vi "Init.vi"(4 "Interlock message (\" -> Interlock!\")":string=" -> Interlock!", 6 "Name (SHV Name if empty)":string, 7 "Sample Containers SHV (Array!)":variant, 8 "error in (no error)":errorcluster, 9 "Stop Self on IL? (T)":bool=TRUE, 11 "Interlock Sample in":refnum<class "Interlock Sample.lvclass">) -> (0 "error out":errorcluster, 3 "Interlock Sample out":refnum<class "Interlock Sample.lvclass">)   [LabVIEW 2015, in "Interlocks.lvlib" / "Interlock Sample.lvclass"]
uses:
  Interlock Sample.lvclass
  Controls/Sample Container.ctl
  subs/Sample/Sample.lvclass
  Interlock Sample.lvclass/Interlock Sample.ctl
  Interlock/Interlock.lvclass/Interlock.ctl
  Interlock/Interlock.lvclass
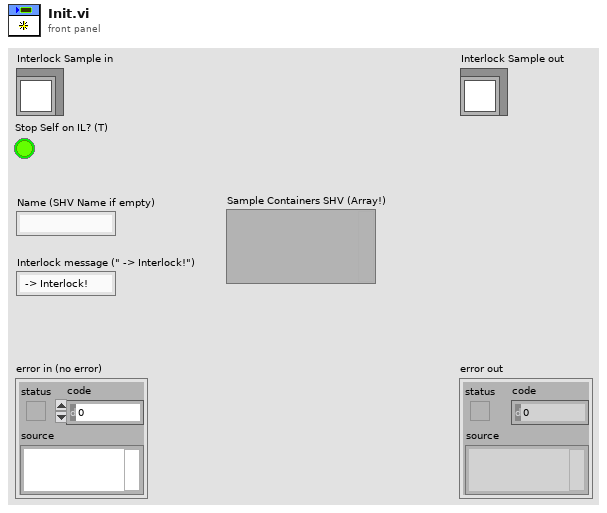
[diagram p1: front panel]
types:
  T1 = typedef "Sample Container.ctl" = cluster{"Sample In":refnum<k21>, "Sample Name":refnum<k21>, "Ti Cathode":refnum<k21>, "SampleQ":refnum<queue>}
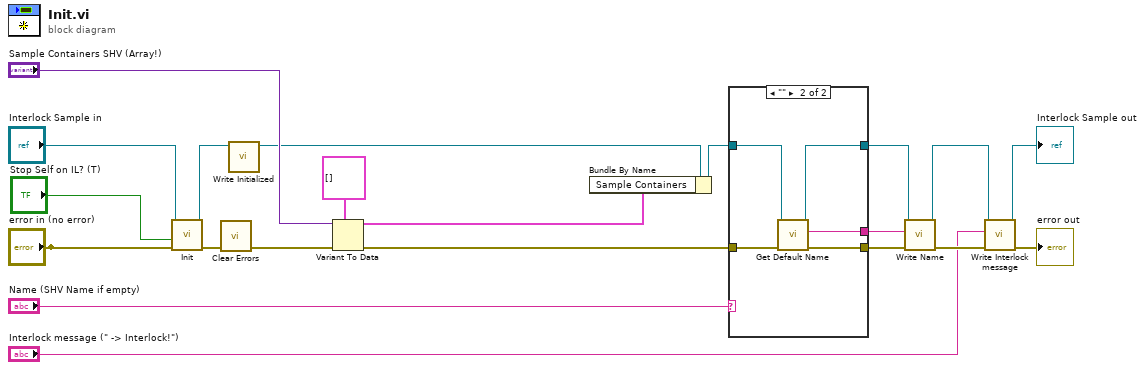
[diagram p0: block diagram]
diagram:
  n1 = call-parent "Init.vi"("error in (no error)"="error in (no error)", "Stop Self on IL? (T)"="Stop Self on IL? (T)", "Interlock in"="Interlock Sample in") -> ("error out"=w7:errorcluster, "Interlock out"=w4:refnum<class "Interlock Sample.lvclass">)  [unwired: 7 in]
  n2 = call <vilib>:"Clear Errors.vi"("error in (no error)"=w7) -> ()  [unwired: 5 in, 2 out]
  n3 = call-dynamic "Write Initialized.vi"("Interlock in"=w4) -> ("Interlock out"=w8:refnum<class "Interlock Sample.lvclass">)  [unwired: 10 in]
  n4 = Variant To Data(error in="error in (no error)", type=T1[] [], Variant="Sample Containers SHV (Array!)") -> (data=w3:T1[], error out=w2:errorcluster)
  n5 = Bundle By Name(cluster=w8, "Sample Containers"=w3) -> (w20:refnum<class "Interlock Sample.lvclass">)
  n6 = case shown="\"\"" "Name (SHV Name if empty)" {
    selector: "Name (SHV Name if empty)" -> [w22 _]
    tunnel: w2 -> [w23 w28]
    tunnel: w20 -> [w21 w27]
    tunnel: [w23 w26] -> w19
    tunnel: [w21 w25] -> w18
    tunnel: [w22 w24] -> w16
    frame "False", Default {
    }
    frame "" {
      n7 = call "Get Default Name.vi"("error in (no error)"=w28, "Interlock Sample in"=w27) -> ("error out"=w26:errorcluster, "Name"=w24:string, "Interlock Sample out"=w25:refnum<class "Interlock Sample.lvclass">)  [unwired: 7 in]
    }
  }
  n8 = call "Write Name.vi"("error in (no error)"=w19, "Name"=w16, "Interlock in"=w18) -> ("error out"=w15:errorcluster, "Interlock out"=w13:refnum<class "Interlock Sample.lvclass">)  [unwired: 7 in]
  n9 = call "Write Interlock message.vi"("error in (no error)"=w15, "Interlock message"="Interlock message (\" -> Interlock!\")", "Interlock in"=w13) -> ("error out"=→"error out":errorcluster, "Interlock out"=→"Interlock Sample out":refnum<class "Interlock Sample.lvclass">)  [unwired: 7 in]
